vi "UA Ring to UA Enum.vi"(1 "OPC UA Data Type Ring":T1=1 items=["Boolean"=1, "SByte"=2, "Byte"=3, "Int16"=4, "UInt16"=5, "Int32"=6, "UInt32"=7, "Int64"=8, "UInt64"=9, "Float"=10, "Double"=11, "String"=12, "DateTime"=13, "ByteString"=15, "Array of Boolean"=101, "Array of SByte"=102, "Array of Byte"=103, "Array of Int16"=104, "Array of UInt16"=105, "Array of Int32"=106, "Array of UInt32"=107, "Array of Int64"=108, "Array of UInt64"=109, "Array of Float"=110, "Array of Double"=111, "Array of String"=112, "Array of DateTime"=113, "Array of ByteString"=115]) -> (0 "OPC Data Type Enum":T2)   [LabVIEW 2014, in "OPC UA Client editor node.lvclass"]
doc: "Convert UA Rint control to Enum control.\n\nRuntime and configuration classes expect ring data type but the table API does not have a ring override. We do this quick type conversion to avoid creating a new class for ring data and changing the connector pane of core libraries."
uses:
  OPC UA Client editor node.lvclass
  OPC UA DataType Enum.ctl
  module/configuration/OPC UA Data Type.ctl
  module/configuration/OPC UA Client configuration.lvclass
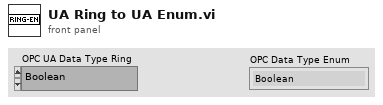
[diagram p1: front panel]
types:
  T1 = typedef "OPC UA Client configuration.lvclass/OPC UA Data Type.ctl" = u16
  T2 = typedef "OPC UA Client editor node.lvclass/OPC UA DataType Enum.ctl" = enum16{"Boolean", "SByte", "Byte", "Int16", "UInt16", "Int32", "UInt32", "Int64", "UInt64", "Float", "Double", "String", "DateTime", "ByteString", "Array of Boolean", "Array of SByte", "Array of Byte", "Array of Int16", "Array of UInt16", "Array of Int32", "Array of UInt32", "Array of Int64", "Array of UInt64", "Array of Float", "Array of Double", "Array of String", "Array of DateTime"}
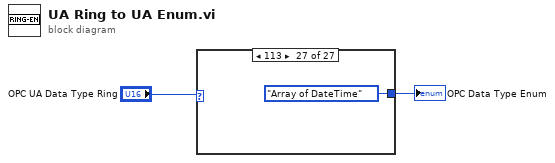
[diagram p0: block diagram]
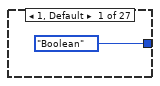
[diagram p2: hidden frame]
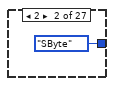
[diagram p3: hidden frame]
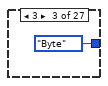
[diagram p4: hidden frame]
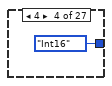
[diagram p5: hidden frame]
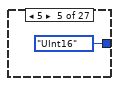
[diagram p6: hidden frame]
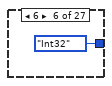
[diagram p7: hidden frame]
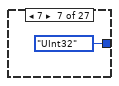
[diagram p8: hidden frame]
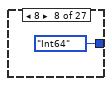
[diagram p9: hidden frame]
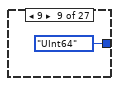
[diagram p10: hidden frame]
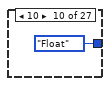
[diagram p11: hidden frame]
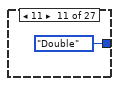
[diagram p12: hidden frame]
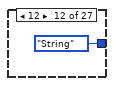
[diagram p13: hidden frame]
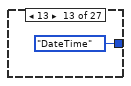
[diagram p14: hidden frame]
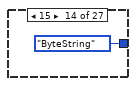
[diagram p15: hidden frame]
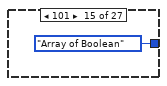
[diagram p16: hidden frame]
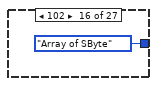
[diagram p17: hidden frame]
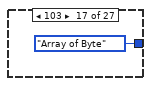
[diagram p18: hidden frame]
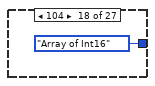
[diagram p19: hidden frame]
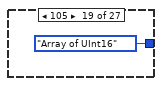
[diagram p20: hidden frame]
diagram:
  n1 = case shown="113" "OPC UA Data Type Ring" {
    tunnel: [OPC_UA_DataType_Enum."Boolean" ("OPC Data Type Enum") OPC_UA_DataType_Enum."SByte" ("OPC Data Type Enum") OPC_UA_DataType_Enum."Byte" ("OPC Data Type Enum") OPC_UA_DataType_Enum."Int16" ("OPC Data Type Enum") OPC_UA_DataType_Enum."UInt16" ("OPC Data Type Enum") OPC_UA_DataType_Enum."Int32" ("OPC Data Type Enum") OPC_UA_DataType_Enum."UInt32" ("OPC Data Type Enum") OPC_UA_DataType_Enum."Int64" ("OPC Data Type Enum") OPC_UA_DataType_Enum."UInt64" ("OPC Data Type Enum") OPC_UA_DataType_Enum."Float" ("OPC Data Type Enum") OPC_UA_DataType_Enum."Double" ("OPC Data Type Enum") OPC_UA_DataType_Enum."String" ("OPC Data Type Enum") OPC_UA_DataType_Enum."DateTime" ("OPC Data Type Enum") OPC_UA_DataType_Enum."ByteString" ("OPC Data Type Enum") OPC_UA_DataType_Enum."Array of Boolean" ("OPC Data Type Enum") OPC_UA_DataType_Enum."Array of SByte" ("OPC Data Type Enum") OPC_UA_DataType_Enum."Array of Byte" ("OPC Data Type Enum") OPC_UA_DataType_Enum."Array of Int16" ("OPC Data Type Enum") OPC_UA_DataType_Enum."Array of UInt16" ("OPC Data Type Enum") OPC_UA_DataType_Enum."Array of Int32" ("OPC Data Type Enum") OPC_UA_DataType_Enum."Array of UInt32" ("OPC Data Type Enum") OPC_UA_DataType_Enum."Array of Int64" ("OPC Data Type Enum") OPC_UA_DataType_Enum."Array of UInt64" ("OPC Data Type Enum") OPC_UA_DataType_Enum."Array of Float" ("OPC Data Type Enum") OPC_UA_DataType_Enum."Array of Double" ("OPC Data Type Enum") OPC_UA_DataType_Enum."Array of String" ("OPC Data Type Enum") OPC_UA_DataType_Enum."Array of DateTime" ("OPC Data Type Enum")] -> w1
    frame 1, Default {
    }
    frame 2 {
    }
    frame 3 {
    }
    frame 4 {
    }
    frame 5 {
    }
    frame 6 {
    }
    frame 7 {
    }
    frame 8 {
    }
    frame 9 {
    }
    frame 10 {
    }
    frame 11 {
    }
    frame 12 {
    }
    frame 13 {
    }
    frame 15 {
    }
    frame 101 {
    }
    frame 102 {
    }
    frame 103 {
    }
    frame 104 {
    }
    frame 105 {
    }
    frame 106 {
    }
    frame 107 {
    }
    frame 108 {
    }
    frame 109 {
    }
    frame 110 {
    }
    frame 111 {
    }
    frame 112 {
    }
    frame 113 {
    }
  }
  "OPC Data Type Enum" <- w1
